vi "CreateWheelfileArray.vi"(8 "error in (no error)":errorcluster, 11 "Wheelfile":string) -> (0 "error out":errorcluster, 3 "Wheelfile Array":string[][](array[string]))   [LabVIEW 2013]
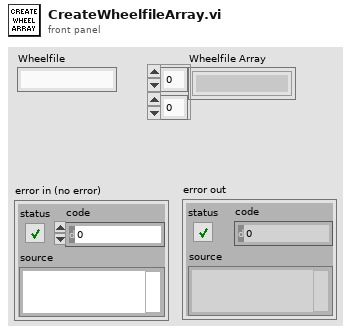
[diagram p1: front panel]
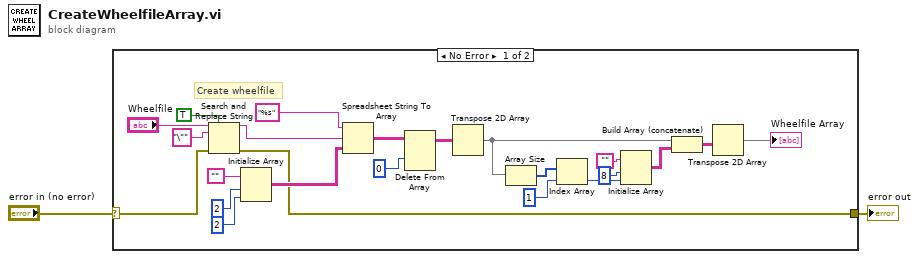
[diagram p0: block diagram]
diagram:
  n1 = case shown="No Error" "error in (no error)" {
    selector: "error in (no error)" -> [w4 w26]
    tunnel: [w3 w26] -> w1
    frame No Error {
      # "Create wheelfile"
      n2 = Search and Replace String(replace all?=TRUE ("replace all? (F)"), input string="Wheelfile", search string="\"", error in=w4) -> (result string=w21:string, error out=w3:errorcluster)  [unwired: 6 out]
      n3 = Initialize Array("" ("format string"), 2 ("dimension size"), 2 ("dimension size")) -> (w9:string[][])
      n4 = Spreadsheet String To Array(format string="%s", spreadsheet string=w21, array type (2D Dbl)=w9) -> (array=w11:string[][])  [unwired: 1 out]
      n5 = Delete From Array(array=w11, index (row)=0) -> (array with subset deleted=w16:string[][])  [unwired: 2 in, 1 out]
      n6 = Transpose 2D Array(2D array=w16) -> (transposed array=w17:string[][])
      n7 = Array Size(array=w17) -> (size(s)=w13:i32[])
      n8 = Index Array(array=w13, index=1) -> (element=w19:i32)
      n9 = Initialize Array("", 8 ("dimension size"), w19) -> (w15:string[][])
      n10 = Build Array (concatenate)(w17, w15) -> (w18:string[][])
      n11 = Transpose 2D Array(2D array=w18) -> (transposed array=→"Wheelfile Array":string[][])
    }
    frame Error {
    }
  }
  "error out" <- w1
